vi "NS_SetProperty.vi"(8 "Error In":errorcluster, 10 "Property":bool, 11 "object in":refnum<class "NativeSubTemplate_4x4x4.lvclass">) -> (0 "Error Out":errorcluster, 3 "object out":refnum<class "NativeSubTemplate_4x4x4.lvclass">)   [LabVIEW 2020, in "NativeSubTemplate_4x4x4.lvclass"]
uses:
  NativeSubTemplate_4x4x4.lvclass
  NativeSubTemplate_4x4x4.lvclass/NativeSubTemplate_4x4x4.ctl
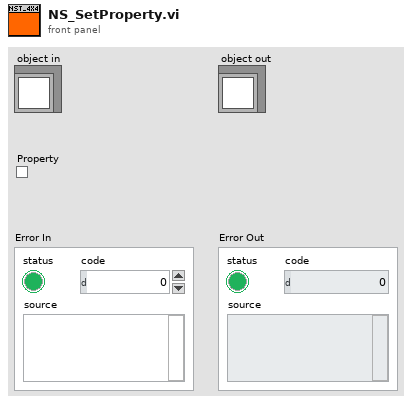
[diagram p1: front panel]
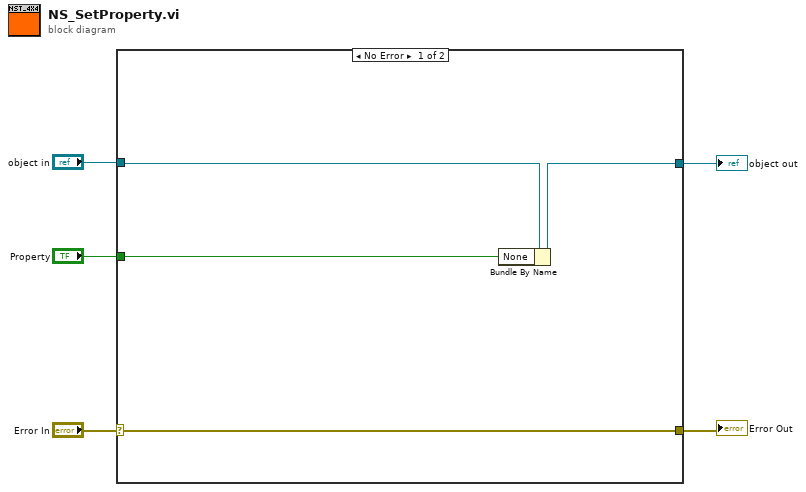
[diagram p0: block diagram]
diagram:
  n1 = case shown="No Error" "Error In" {
    selector: "Error In" -> [w8 w11]
    tunnel: [w8 w11] -> w4
    tunnel: [w6 w10] -> w2
    tunnel: "object in" -> [w7 w10]
    tunnel: "Property" -> [w9 _]
    frame No Error {
      n2 = Bundle By Name(cluster=w7, "None"=w9) -> (w6:refnum<class "NativeSubTemplate_4x4x4.lvclass">)
    }
    frame Error {
    }
  }
  "Error Out" <- w4
  "object out" <- w2
